vi "zmq_send_multi.vi"(3 "error in":errorcluster, 4 "parts":string[](array[string]), 5 "socket in":refnum<class "zmq_socket.lvclass">) -> (0 "error out":errorcluster, 2 "socket out":refnum<class "zmq_socket.lvclass">)   [LabVIEW 2020, in "zeromq.lvlib" / "zmq_socket.lvclass"]
doc: "Sends a multi-component message corresponding to the elements of <b>parts</b> through the socket."
uses:
  zmq_socket.lvclass
  zmq_socket.lvclass/zmq_socket.ctl
  Error Cluster From Error Code.vi
  zeromq.lvlib
panel:
  # "ØMQ"
  # "labview"
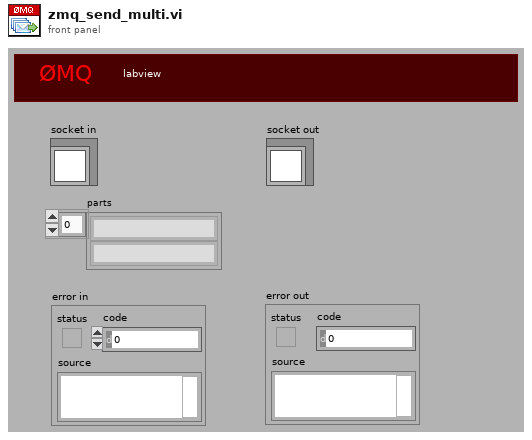
[diagram p1: front panel]
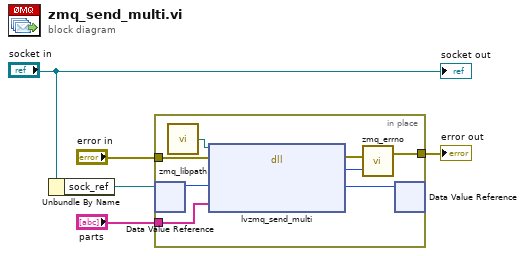
[diagram p0: block diagram]
diagram:
  n1 = Unbundle By Name("socket in") -> ("sock_ref"=w1:refnum<data-value>)
  n2 = in-place {
    in-place-border: "parts" -> [w11]
    in-place-border: "error in" -> [w10]
    in-place-border: [w9] -> w3
    n3 = in-place-dvr #1(w1) -> (w8:u64)  [unwired: 1 out]
    n4 = call "zmq_libpath.vi"() -> ("path"=w6:path)
    n5 = dll-call lib="?" fn="lvzmq_send_multi" ("zmq_labview.dll:lvzmq_socket")(path in=w6, error in=w10, "sock_obj"=w8, "data"=w11) -> (error out=w13:errorcluster, "return type"=w12:i32, "sock_obj"=w7:u64)  [unwired: 2 in, 1 out]
    n6 = call "zmq_errno.vi"("retval"=w12, "error in"=w13) -> ("error out"=w9:errorcluster)  [unwired: 1 out]
    n7 = in-place-dvr #1(w7) -> ()  [unwired: 2 out]
  }
  "error out" <- w3
  "socket out" <- "socket in"
